vi "set_out.vi"(11 "Outputs":T1) -> ()   [LabVIEW 2013]
uses:
  outputs.ctl
  drive/drive_outputs.ctl
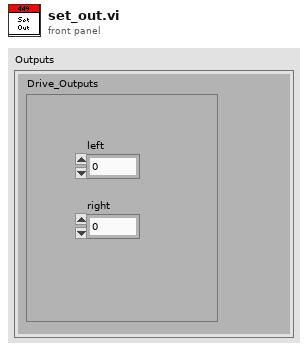
[diagram p1: front panel]
types:
  T1 = typedef "outputs.ctl" = cluster{"Drive_Outputs":T2}
  T2 = typedef "drive_outputs.ctl" = cluster{"left":dbl, "right":dbl}
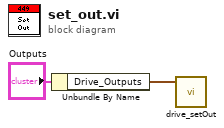
[diagram p0: block diagram]
diagram:
  n1 = Unbundle By Name("Outputs") -> ("Drive_Outputs"=w1:T2)
  n2 = call "drive_setOut.vi"("Drive_Outputs"=w1) -> ()  [unwired: 11 in]
